vi "B_doThis.vi"(10 "input":dbl) -> (2 "output":dbl)   [LabVIEW 2016, in "LibB.lvlib"]
uses:
  LibB.lvlib
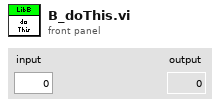
[diagram p1: front panel]
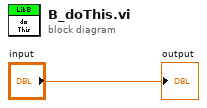
[diagram p0: block diagram]
diagram:
  "output" <- "input"
